vi "Init MCL.vi"(8 "Error In":errorcluster, 11 "MCL Reference":refnum<vi>) -> (0 "Error Out":errorcluster)   [LabVIEW 2023, in "Error Manager.lvlib" / "MCL.lvclass"]
doc: "Blank VI with error handling."
uses:
  <vilib>/Utility/miscctls.llb/LVBoundsTypeDef.ctl
  <vilib>/Utility/miscctls.llb/LVRowAndColumnTypeDef.ctl
  <vilib>/Utility/miscctls.llb/LVRowAndColumnUnsignedTypeDef.ctl
  MCL.lvclass
  MCL.lvclass/MCL.ctl
panel:
  out "Row Sizes":T1[](array[typedef])
  # "Input\nInputs to the VI"
  # "Development\nControls or indicators that are useful for development or testing, but which are not outputs of the VI."
  # "Output\nOutputs of the VI"
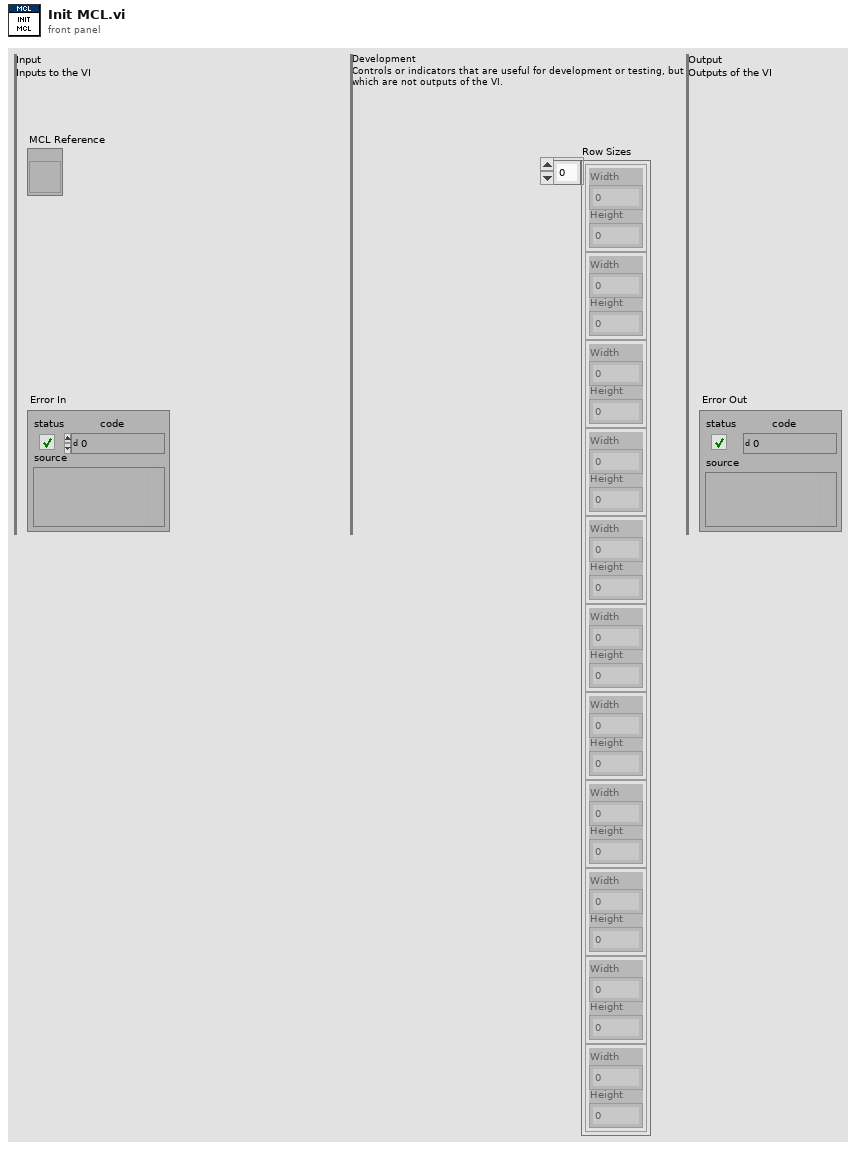
[diagram p1: front panel]
types:
  T1 = typedef "LVBoundsTypeDef.ctl" = cluster{"Width":u32, "Height":u32}
  T2 = typedef "LVRowAndColumnTypeDef.ctl" = cluster{"Row":i32, "Column":i32}
  T3 = typedef "LVRowAndColumnUnsignedTypeDef.ctl" = cluster{"Row":u32, "Column":u32}
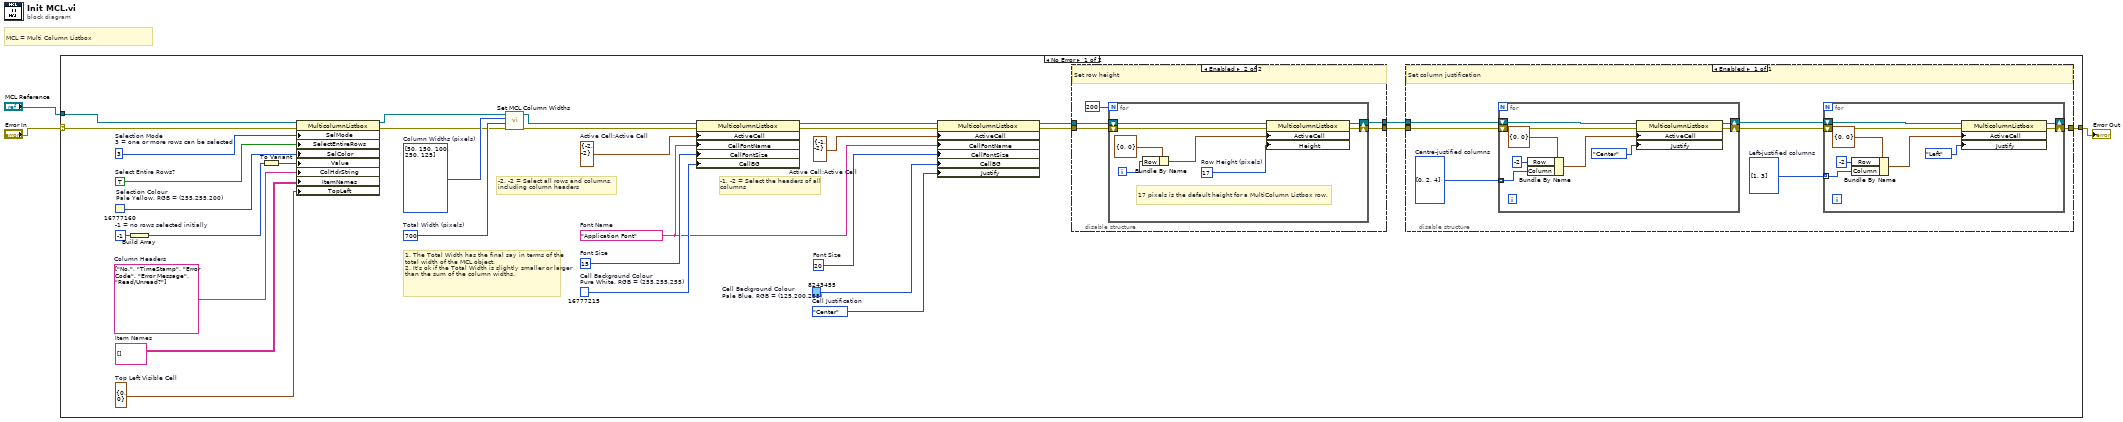
[diagram p0: block diagram]
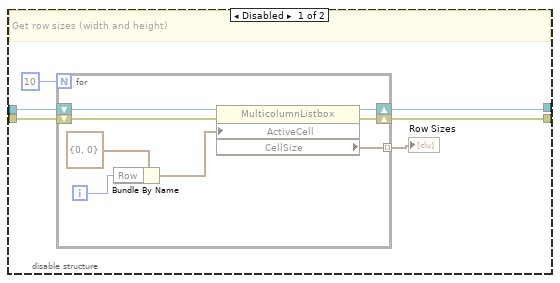
[diagram p2: hidden frame]
diagram:
  # "MCL = Multi Column Listbox"
  n1 = case shown="No Error" "Error In" {
    selector: "Error In" -> [w35 w88]
    tunnel: "MCL Reference" -> [w19 _]
    tunnel: [w5 w88] -> w1
    frame No Error {
      w9 = enum16{"Left", "Center", "Right"}."Center"  # Cell Justification
      w10 = u32 8243455  # Cell Background Colour Pale Blue, RGB = (125,200,255)
      w11 = T3 {"Row"=0, "Column"=0}  # Top Left Visible Cell
      w16 = -1  # -1 = no rows selected initially
      w17 = string[][] []  # Item Names
      w21 = 3  # Selection Mode 3 = one or more rows can be selected
      w12 = u32 16777160  # Selection Colour Pale Yellow, RGB = (255,255,200)
      w13 = TRUE  # Select Entire Rows?
      w23 = u32 20  # Font Size
      w25 = T2 {"Row"=-1, "Column"=-2}  # Active Cell:Active Cell
      w28 = u32 16777215  # Cell Background Colour Pure White, RGB = (255,255,255)
      w29 = u32 15  # Font Size
      w24 = "Application Font"  # Font Name
      w30 = T2 {"Row"=-2, "Column"=-2}  # Active Cell:Active Cell
      w33 = u32 700  # Total Width (pixels)
      w34 = u32[] [50, 150, 100, 250, 125]  # Column Widths (pixels)
      w18 = string[] ["No.", "TimeStamp", "Error Code", "Error Message", "Read/Unread?"]  # Column Headers
      # "-1, -2 = Select the headers of all columns"
      # "-2, -2 = Select all rows and columns, including column headers"
      # "1. The Total Width has the final say in terms of the total width of the MCL object.\n2. It's ok if the Total Width is slightly smaller or larger than the sum of the column widths."
      n2 = Build Array(w16) -> (w15:i32[])
      n3 = To Variant(anything=w15) -> (Variant=w14:variant)
      n4 = property class="MulticolumnListbox"(reference=w19, error in=w35, "SelMode"=w21, "SelectEntireRows"=w13, "SelColor"=w12, "Value"=w14, "ColHdrString"=w18, "ItemNames"=w17, "TopLeft"=w11) -> (reference out=w20:refnum<vi>, error out=w22:errorcluster)
      n5 = call "Set MCL Column Widths.vi"("error in (no error)"=w22, "Total Width (pixels)"=w33, "Column Widths (pixels)"=w34, "MCL Ref In"=w20) -> ("error out"=w31:errorcluster, "MCL Ref Out"=w32:refnum<vi>)  [unwired: 6 in]
      n6 = property class="MulticolumnListbox"(reference=w32, error in=w31, "ActiveCell"=w30, "CellFontName"=w24, "CellFontSize"=w29, "CellBG"=w28) -> (reference out=w26:refnum<vi>, error out=w27:errorcluster)
      n7 = property class="MulticolumnListbox"(reference=w26, error in=w27, "ActiveCell"=w25, "CellFontName"=w24, "CellFontSize"=w23, "CellBG"=w10, "Justify"=w9) -> (reference out=w8:refnum<vi>, error out=w7:errorcluster)
      n8 = disable-structure shown="Enabled" {
        disable-tunnel: w8 -> [w66 w79]
        disable-tunnel: w7 -> [w65 w78]
        disable-tunnel: [w64 w77] -> w6
        disable-tunnel: [w61 w75] -> w4
        frame Disabled {
          # "Get row sizes (width and height)"
          n9 = for {
            N: 10 -> [_]
            shift-right: [w71] -> w64
            shift-left: w65 -> [w72]
            tunnel: [w68] -> w62 mode=indexing
            shift-right: [w67] -> w61
            shift-left: w66 -> [w74]
            i -> [w69]
            n10 = Bundle By Name(cluster=T2 {"Row"=0, "Column"=0} ("Active Cell:Active Cell"), "Row"=w69) -> (w70:T2)
            n11 = property class="MulticolumnListbox"(reference=w74, error in=w72, "ActiveCell"=w70) -> (reference out=w67:refnum<vi>, error out=w71:errorcluster, "CellSize"=w68:T1)
          }
          "Row Sizes" <- w62
        }
        frame Enabled {
          # "Set row height"
          n12 = for {
            N: 200 -> [_]
            shift-right: [w84] -> w77
            shift-left: w78 -> [w85]
            shift-right: [w80] -> w75
            shift-left: w79 -> [w87]
            i -> [w82]
            w81 = u32 17  # Row Height (pixels)
            # "17 pixels is the default height for a MultiColumn Listbox row."
            n13 = Bundle By Name(cluster=T2 {"Row"=0, "Column"=0} ("Active Cell:Active Cell"), "Row"=w82) -> (w83:T2)
            n14 = property class="MulticolumnListbox"(reference=w87, error in=w85, "ActiveCell"=w83, "Height"=w81) -> (reference out=w80:refnum<vi>, error out=w84:errorcluster)
          }
        }
      }
      n15 = disable-structure shown="Enabled" {
        disable-tunnel: w4 -> [w42]
        disable-tunnel: w6 -> [w41]
        disable-tunnel: [w38] -> w5
        frame Enabled {
          w37 = i32[] [1, 3]  # Left-justified columns
          w40 = i32[] [0, 2, 4]  # Centre-justified columns
          # "Set column justification"
          n16 = for {
            shift-right: [w48] -> w39
            shift-left: w41 -> [w49]
            tunnel: w40 -> [w45] mode=indexing
            shift-right: [w43] -> w36
            shift-left: w42 -> [w51]
            n17 = Bundle By Name(cluster=T2 {"Row"=0, "Column"=0} ("Active Cell:Active Cell"), "Row"=-2, "Column"=w45) -> (w47:T2)
            n18 = property class="MulticolumnListbox"(reference=w51, error in=w49, "ActiveCell"=w47, "Justify"=enum16{"Left", "Center", "Right"}."Center" ("Active Cell:Cell Justification")) -> (reference out=w43:refnum<vi>, error out=w48:errorcluster)
          }
          n19 = for {
            shift-right: [w57] -> w38
            shift-left: w39 -> [w58]
            tunnel: w37 -> [w54] mode=indexing
            shift-right: [w52] -> _
            shift-left: w36 -> [w60]
            n20 = Bundle By Name(cluster=T2 {"Row"=0, "Column"=0} ("Active Cell:Active Cell"), "Row"=-2, "Column"=w54) -> (w56:T2)
            n21 = property class="MulticolumnListbox"(reference=w60, error in=w58, "ActiveCell"=w56, "Justify"=enum16{"Left", "Center", "Right"}."Left" ("Active Cell:Cell Justification")) -> (reference out=w52:refnum<vi>, error out=w57:errorcluster)
          }
        }
      }
    }
    frame Error {
    }
  }
  "Error Out" <- w1
